vi "xml.string.vi"(10 "Value":variant, 11 "MsgSerializer.XML in":refnum<class "MsgSerializer.XML.lvclass">) -> (3 "string":string)   [LabVIEW 2013, in "Caraya.lvlib" / "MsgSerializer.XML.lvclass"]
uses:
  MsgSerializer.XML.lvclass
  MsgSerializer.XML.lvclass/MsgSerializer.XML.ctl
  MsgSerializer/MsgSerializer.lvclass/MsgSerializer.ctl
  MsgSerializer/MsgSerializer.lvclass
  <vilib>/Utility/VariantDataType/VariantType.lvlib
  Caraya.lvlib
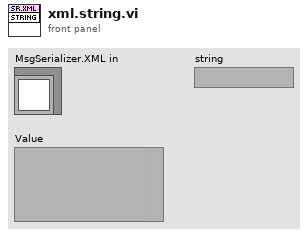
[diagram p1: front panel]
types:
  T1 = typedef "VariantType.lvlib/Type.ctl" = enum8{"Invalid Type", "Void", "I8", "I16", "I32", "I64", "U8", "U16", "U32", "U64", "Single Float", "Double Float", "Extended Float", "Single Complex", "Double Complex", "Extended Complex", "Enum U8", "Enum U16", "Enum U32", "Enum U64", "Single Float With Unit", "Double Float With Unit", "Extended Float With Unit", "Single Complex with Unit", "Double Complex with Unit", "Extended Complex with Unit", "Boolean", "String", "Path", "Picture", "Tag", "Array", "Cluster", "Variant", "LV Variant", "Waveform", "Timestamp", "Digital Waveform", "Digital Data", "ExpressData", "Refnum", "External Data", "VI", "Poly VI", "LabVIEW Class Instance", "Fixed Point"}
  T2 = typedef "Caraya.lvlib/MsgSerializer.XML.lvclass/format -- enum.ctl" = enum16{"value", "tag", "property"}
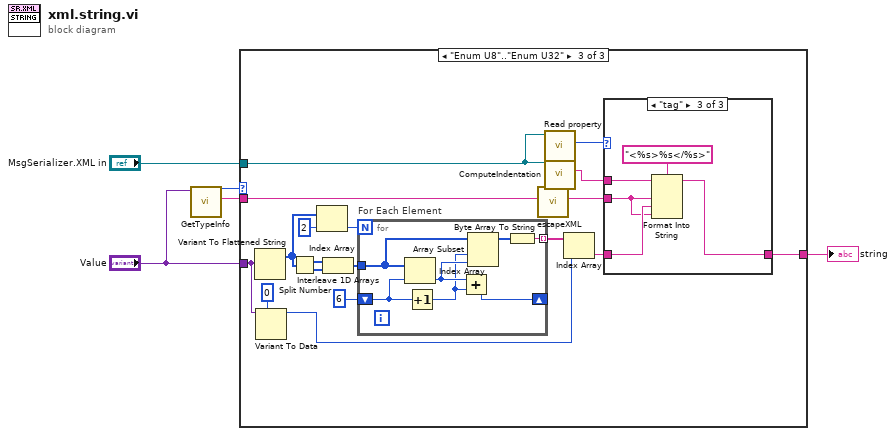
[diagram p0: block diagram]
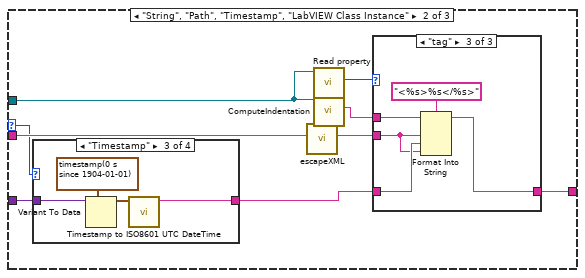
[diagram p3: hidden frame]
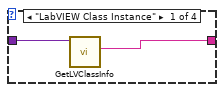
[diagram p4: hidden frame]
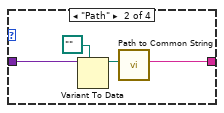
[diagram p5: hidden frame]
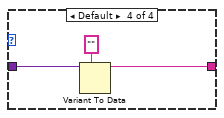
[diagram p6: hidden frame]
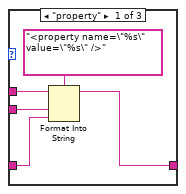
[diagram p7: hidden frame]
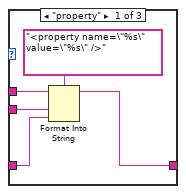
[diagram p9: hidden frame]
diagram:
  n1 = call <vilib>:"GetTypeInfo.vi"("Variant"="Value") -> ("Name"=w4:string, "Type Enum"=w1:T1)  [unwired: 6 in, 3 out]
  n2 = case shown="\"Enum U8\"..\"Enum U32\"" w1 {
    selector: w1 -> [_ w7 _]
    tunnel: "Value" -> [_ w8 w39]
    tunnel: w4 -> [_ w12 w54]
    tunnel: "MsgSerializer.XML in" -> [_ w10 w52]
    tunnel: [_ w9 w51] -> w2
    frame Default {
    }
    frame "String", "Path", "Timestamp", "LabVIEW Class Instance" {
      n3 = case shown="\"Timestamp\"" w7 {
        tunnel: w8 -> [w16 w18 w21 w26]
        tunnel: [w15 w17 w22 w25] -> w6
        frame "LabVIEW Class Instance" {
          n4 = call <vilib>:"GetLVClassInfo.vi"("Variant"=w16) -> ("LV Class File Name"=w15:string)  [unwired: 8 in, 2 out]
        }
        frame "Path" {
          n5 = Variant To Data(type=path "", Variant=w18) -> (data=w19:path)  [unwired: 1 in, 1 out]
          n6 = call "Path to Common String.vi"("specific path"=w19) -> ("common path"=w17:string)  [unwired: 10 in]
        }
        frame "Timestamp" {
          n7 = Variant To Data(type=timestamp(0 s since 1904-01-01) ("current time"), Variant=w21) -> (data=w23:timestamp)  [unwired: 1 in, 1 out]
          n8 = call <vilib>:"Timestamp to ISO8601 UTC DateTime.vi"("Timestamp (now)"=w23) -> ("ISO8601 UTC DateTime"=w22:string)  [unwired: 10 in]
        }
        frame Default {
          n9 = Variant To Data(type="", Variant=w26) -> (data=w25:string)  [unwired: 1 in, 1 out]
        }
      }
      n10 = call "escapeXML.vi"("Input String"=w12) -> ("XML-escaped String"=w13:string)  [unwired: 10 in]
      n11 = call "Read property.vi"("MsgSerializer.XMLProperty in"=w10) -> ("format"=w14:T2)  [unwired: 9 in, 1 out]
      n12 = call "ComputeIndentation.vi"("MsgSerializer in"=w10) -> ("indentation"=w11:string)  [unwired: 10 in]
      n13 = case shown="\"tag\"" w14 {
        tunnel: w6 -> [w31 w33 w37]
        tunnel: [w30 w33 w34] -> w9
        tunnel: w11 -> [w28 _ w36]
        tunnel: w13 -> [w29 _ w35]
        frame "property" {
          n14 = Format Into String(format string="<property name=\"%s\" value=\"%s\" />" ("name"), initial string=w28, w29, w31) -> (resulting string=w30:string)  [unwired: 1 in, 1 out]
        }
        frame "value" {
        }
        frame "tag" {
          n15 = Format Into String(format string="<%s>%s</%s>" ("name"), initial string=w36, w35, w37, w35) -> (resulting string=w34:string)  [unwired: 1 in, 1 out]
        }
      }
    }
    frame "Enum U8".."Enum U32" {
      n16 = Variant To Flattened String(Variant=w39) -> (1:w42:i16[])  [unwired: 1 out]
      n17 = Variant To Data(type=u32 0, Variant=w39) -> (data=w41:u32)  [unwired: 1 in, 1 out]
      n18 = Split Number(x=w42) -> (hi(x)=w47:u8[], lo(x)=w46:u8[])
      n19 = Index Array(array=w42, index=2) -> (element=w49:i16)
      n20 = Interleave 1D Arrays(w47, w46) -> (w45:u8[])
      n21 = for "For Each Element" {
        N: w49 -> [_]
        shift-right: [w60] -> _
        shift-left: 6 ("index") -> [w63]
        tunnel: w45 -> [w61]
        tunnel: [w58] -> w43 mode=indexing
        n22 = Index Array(array=w61, index=w63) -> (element=w59:u8)
        n23 = Increment(x=w63) -> (x+1=w57:i32)
        n24 = Add(x=w59, y=w57) -> (x+y=w60:i32)
        n25 = Array Subset(array=w61, index=w57, length=w59) -> (w62:u8[])
        n26 = Byte Array To String(unsigned byte array=w62) -> (string=w58:string)
      }
      n27 = call "escapeXML.vi"("Input String"=w54) -> ("XML-escaped String"=w55:string)  [unwired: 10 in]
      n28 = call "Read property.vi"("MsgSerializer.XMLProperty in"=w52) -> ("format"=w56:T2)  [unwired: 9 in, 1 out]
      n29 = call "ComputeIndentation.vi"("MsgSerializer in"=w52) -> ("indentation"=w53:string)  [unwired: 10 in]
      n30 = Index Array(array=w43, index=w41) -> (element=w40:string)
      n31 = case shown="\"tag\"" w56 {
        tunnel: w40 -> [w67 w69 w73]
        tunnel: [w66 w69 w70] -> w51
        tunnel: w53 -> [w64 _ w72]
        tunnel: w55 -> [w65 _ w71]
        frame "property" {
          n32 = Format Into String(format string="<property name=\"%s\" value=\"%s\" />" ("name"), initial string=w64, w65, w67) -> (resulting string=w66:string)  [unwired: 1 in, 1 out]
        }
        frame "value" {
        }
        frame "tag" {
          n33 = Format Into String(format string="<%s>%s</%s>" ("name"), initial string=w72, w71, w73, w71) -> (resulting string=w70:string)  [unwired: 1 in, 1 out]
        }
      }
    }
  }
  "string" <- w2
